vi "LWXPS_MultipleAxesPVTVerificationResultGet.vi"(1 "XPS Reference IN":refnum<k24>, 2 "Positioner Name":string, 4 "LabVIEW error IN":errorcluster) -> (10 "XPS Reference OUT":refnum<k24>, 12 "Returned error code":i32, 13 "LabVIEW error OUT":errorcluster, 14 "Trajectory File Name":string, 15 "Minimum Position":dbl, 16 "Maximum Position":dbl, 17 "Maximum Velocity":dbl, 18 "Maximum Acceleration":dbl, 19 "XPS Error String":string)   [LabVIEW 2014]
uses:
  D:/XPSQ8_LabView_Library/Development/Source/Dll/Newport.XPS.CommandInterface.dll
  Dll/Newport.XPS.CommandInterface.dll
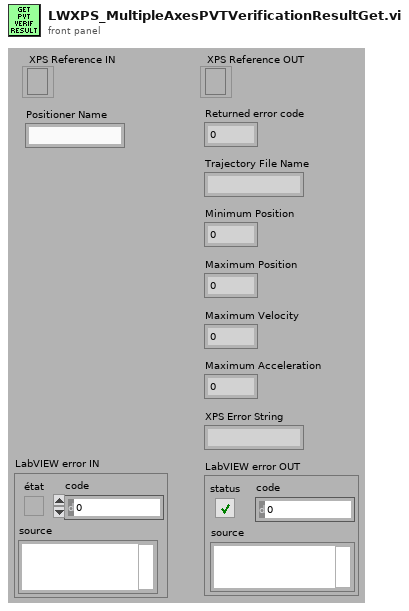
[diagram p1: front panel]
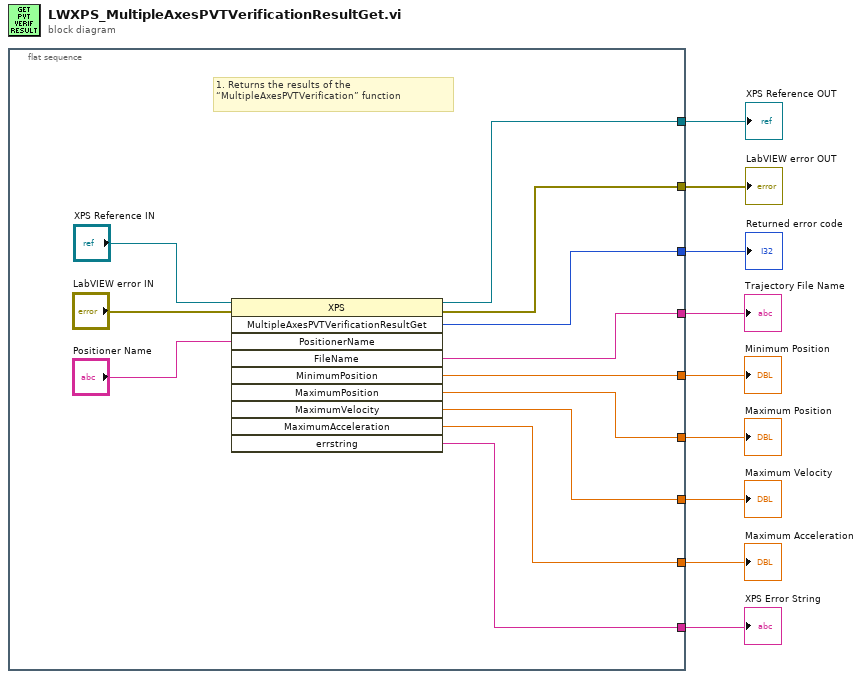
[diagram p0: block diagram]
diagram:
  n1 = flat-sequence {
    tunnel: [w18] -> w8
    tunnel: [w19] -> w9
    tunnel: [w17] -> w7
    tunnel: [w16] -> w6
    tunnel: [w14] -> w4
    tunnel: [w11] -> w1
    tunnel: [w13] -> w3
    tunnel: [w12] -> w2
    tunnel: [w15] -> w5
    frame #0 {
      # "1. Returns the results of the “MultipleAxesPVTVerification” function"
      n2 = invoke class="XPS" method="MultipleAxesPVTVerificationResultGet"(reference="XPS Reference IN", error in="LabVIEW error IN", "PositionerName"="Positioner Name") -> (reference out=w18:refnum<k24>, error out=w19:errorcluster, "MultipleAxesPVTVerificationResultGet"=w17:i32, "FileName"=w16:string, "MinimumPosition"=w15:dbl, "MaximumPosition"=w14:dbl, "MaximumVelocity"=w13:dbl, "MaximumAcceleration"=w12:dbl, "errstring"=w11:string)  [unwired: 7 in, 1 out]
    }
  }
  "XPS Reference OUT" <- w8
  "LabVIEW error OUT" <- w9
  "XPS Error String" <- w1
  "Returned error code" <- w7
  "Trajectory File Name" <- w6
  "Minimum Position" <- w5
  "Maximum Position" <- w4
  "Maximum Velocity" <- w3
  "Maximum Acceleration" <- w2
